vi "Event_ball_out.vi"(8 "error in (no error)":errorcluster, 10 "Game in":refnum<class "Game.lvclass">, 11 "Events in":refnum<class "Events.lvclass">) -> (0 "error out":errorcluster, 3 "Events out":refnum<class "Events.lvclass">)   [LabVIEW 2018, in "Events.lvclass"]
uses:
  Events.lvclass
  Game_class/Game.lvclass
  Game_class/Game.lvclass/Game.ctl
  Object_class/Object.lvclass/Object.ctl
  Events.lvclass/Events.ctl
  Game_class/Read FieldRef.vi
  Game_class/Read BallRef.vi
  Object_class/Read x.vi
  Object_class/Read y.vi
  Write ball_out.vi
  Ball_class/Ball.lvclass
  C:/Users/Leonardo/Documents/RoboIme/Futebol/SSL/SSL-Phoenix/SSL_AI/Object_class/Object.lvclass
  Field_class/Field.lvclass
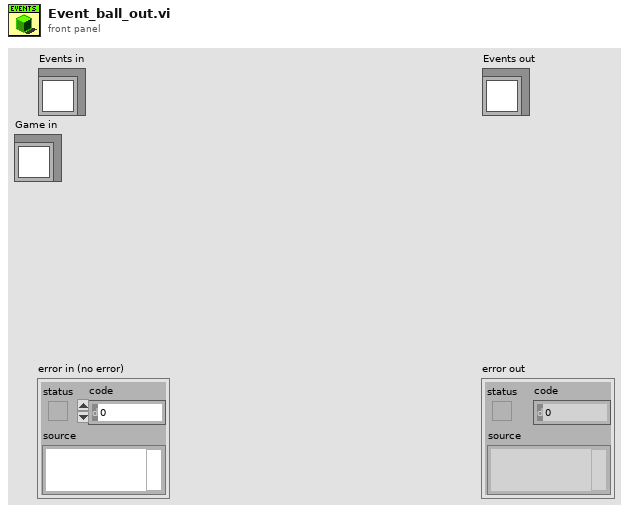
[diagram p1: front panel]
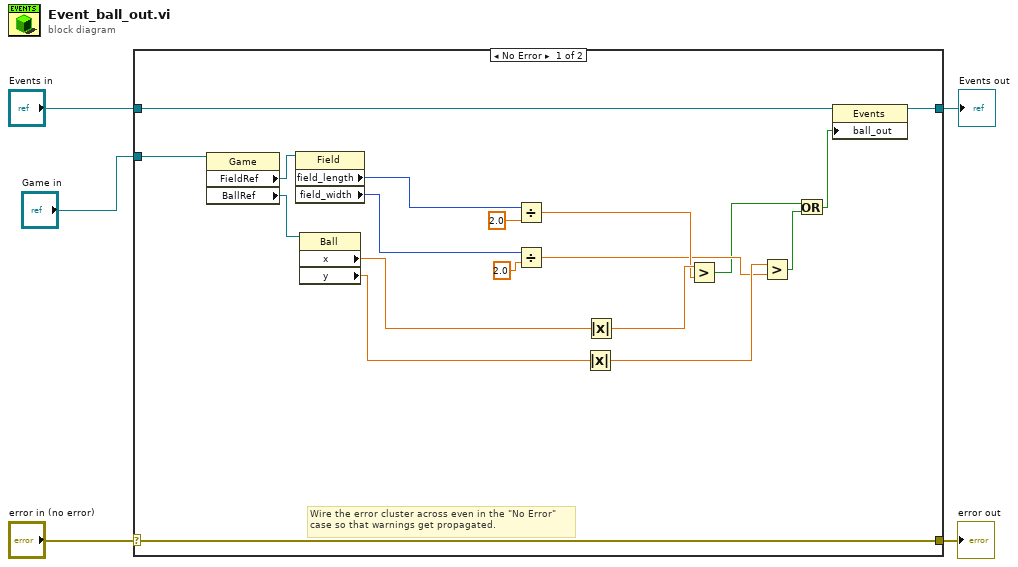
[diagram p0: block diagram]
diagram:
  n1 = case shown="No Error" "error in (no error)" {
    selector: "error in (no error)" -> [w24 w26]
    tunnel: [w24 w26] -> w4
    tunnel: [w7 w25] -> w2
    tunnel: "Events in" -> [w8 w25]
    tunnel: "Game in" -> [w15 _]
    frame No Error {
      # "Wire the error cluster across even in the \"No Error\"\ncase so that warnings get propagated."
      n2 = property class="Game"(reference=w15) -> ("FieldRef"=w14:refnum<class "Field.lvclass">, "BallRef"=w11:refnum<class "Ball.lvclass">)  [unwired: 1 in, 2 out]
      n3 = property class="Field"(reference=w14) -> ("field_length"=w13:i32, "field_width"=w12:i32)  [unwired: 1 in, 2 out]
      n4 = property class="Ball"(reference=w11) -> ("x"=w10:dbl, "y"=w9:dbl)  [unwired: 1 in, 2 out]
      n5 = Divide(x=w13, y=2.0 ("x/y")) -> (x/y=w22:dbl)
      n6 = Divide(x=w12, y=2.0 ("x")) -> (x/y=w20:dbl)
      n7 = Absolute Value(x=w9) -> (abs(x)=w21:dbl)
      n8 = Absolute Value(x=w10) -> (abs(x)=w23:dbl)
      n9 = Greater?(x=w23, y=w22) -> (0:w19:bool)
      n10 = Greater?(x=w21, y=w20) -> (0:w18:bool)
      n11 = Or(x=w19, y=w18) -> (x .or. y?=w6:bool)
      n12 = property class="Events"(reference=w8, "ball_out"=w6) -> (reference out=w7:refnum<class "Events.lvclass">)  [unwired: 1 in, 1 out]
    }
    frame Error {
    }
  }
  "error out" <- w4
  "Events out" <- w2
